vi "DblToStr.vi"(9 "RangeChB":T1(ring) caption="Диапазон \"B\"", 10 "RangeChA":T2(ring) caption="Диапазон \"A\"", 11 "DataDbl":dbl[](array[numeric])=[0.00234, 2.0, 3.0, 4.0]) -> (3 "Out":string[](array[string])=["2.340E-3", "2.000E+0", "3.000E+0", "4.000E+0"])   [LabVIEW 2017]
panel:
  out "final array":string[](array[string])
  in  "Array":string[](array[string])=["%^.3e", "%^.3e", "%^.3f", "%^.3f"]
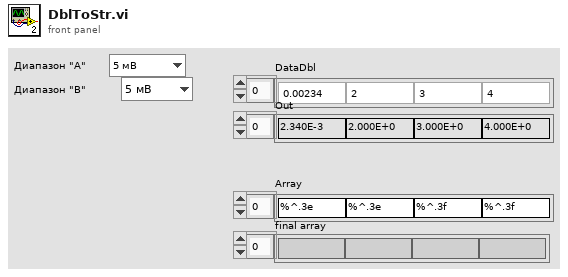
[diagram p1: front panel]
types:
  T1 = enum16{"5 мВ", "10 мВ", "25 мВ", "50 мВ", "100 мВ", "250 мВ", "0,5 В", "1 В", "2,5 В", "5 В", "10 В", "Авто", "Выкл."}
  T2 = enum16{"5 мВ", "10 мВ", "25 мВ", "50 мВ", "100 мВ", "250 мВ", "0,5 В", "1,0 В", "2,5 В", "5 В", "10 В", "Авто", "Выкл."}
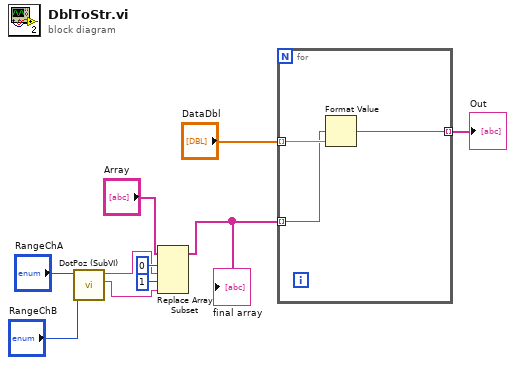
[diagram p0: block diagram]
diagram:
  n1 = call "DotPoz (SubVI).vi"("RangeChB"="RangeChB", "RangeChA"="RangeChA") -> ("Chanal B"=w1:string, "Chanal A"=w2:string)  [unwired: 6 in, 2 out]
  n2 = Replace Array Subset(array="Array", new element #1=w2, index #1=0 ("index"), new element #2=w1, index #2=1 ("index")) -> (w5:string[])
  "final array" <- w5
  n3 = for {
    tunnel: "DataDbl" -> [w13] mode=indexing
    tunnel: w5 -> [w12] mode=indexing
    tunnel: [w11] -> w9 mode=indexing
    n4 = Format Value(format string=w12, value (0)=w13) -> (output string=w11:string)  [unwired: 1 in]
  }
  "Out" <- w9
